vi "c_Load Config Data.vi"() -> (1 "Case Label":T1)   [LabVIEW 2017, in "Settings.lvclass"]
uses:
  Settings.lvclass
  <vilib>/addons/_Workers/Library/Case Label.ctl
  <vilib>/addons/_Workers/Library/Workers.lvlib
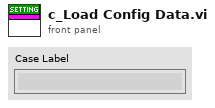
[diagram p1: front panel]
types:
  T1 = typedef "Workers.lvlib/Case Label.ctl" = string
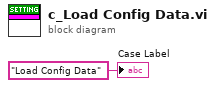
[diagram p0: block diagram]
diagram:
  "Case Label" <- T1 "Load Config Data" ("Case Label")
